vi "智能锁模.vi"() -> ()   [LabVIEW 2017]
panel:
  out "波形图表":dbl[](graph)=[-0.6363858363858363, -0.6363858363858363, -0.6490842490842491, 0.5611721611721612, 0.5142857142857142, 0.4586080586080586, 0.398046398046398, 0.32967032967032966, 0.2564102564102564, 0.1772893772893773, 0.09816849816849817, 0.016117216117216115, -0.06593406593406594, -0.147985347985348, -0.22417582417582418, -0.2993894993894994, -0.3716727716727717, -0.4332112332112332, -0.4918192918192918, -0.5416361416361416, -0.5826617826617827, -0.6148962148962149, -0.6363858363858363, -0.6490842490842491, -0.652014652014652, -0.6422466422466423, -0.6236874236874237, -0.5973137973137973, -0.5582417582417583, -0.5123321123321123, -0.45665445665445664, -0.3941391941391941, -0.32576312576312577, -0.2525030525030525, -0.17533577533577532, -0.09328449328449329, -0.014163614163614164, 0.06788766788766788, 0.14896214896214896, 0.2271062271062271, 0.3023199023199023, 0.3716727716727717, 0.43614163614163615, 0.4937728937728938, 0.5445665445665445, 0.5846153846153846, 0.6178266178266179, 0.6383394383394383, 0.652014652014652, 0.652014652014652, 0.6432234432234433, 0.6266178266178266, 0.5982905982905983, 0.5592185592185592, 0.5142857142857142, 0.45958485958485956, 0.39706959706959705, 0.3286935286935287, 0.2554334554334554, 0.17826617826617827, 0.09816849816849817, 0.017094017094017096, -0.06593406593406594, -0.147008547008547, -0.22612942612942613, -0.30036630036630035, -0.3716727716727717, -0.4341880341880342, -0.4918192918192918, -0.5426129426129426, -0.5836385836385837, -0.613919413919414, -0.6373626373626373, -0.6481074481074481, -0.652014652014652, -0.6442002442002442, -0.6246642246642247, -0.5963369963369963, -0.5572649572649573, -0.5103785103785103, -0.45567765567765567, -0.3941391941391941, -0.32673992673992674, -0.2515262515262515, -0.17631257631257632, -0.09523809523809523, -0.013186813186813187, 0.06788766788766788, 0.147985347985348, 0.2271062271062271, 0.3023199023199023, 0.3716727716727717, 0.43614163614163615, 0.49572649572649574, 0.5435897435897435, 0.5846153846153846, 0.6178266178266179, 0.6383394383394383, 0.652014652014652, 0.652991452991453, 0.6461538461538462, 0.6266178266178266, 0.5992673992673992, 0.5601953601953602, 0.5123321123321123, 0.45958485958485956, 0.39706959706959705, 0.32967032967032966, 0.25445665445665444, 0.1772893772893773, 0.0971916971916972, 0.016117216117216115, -0.06691086691086691, -0.147008547008547, -0.22515262515262516, -0.30036630036630035, -0.3706959706959707, -0.4341880341880342, -0.4908424908424908, -0.5416361416361416, -0.5816849816849817, -0.6148962148962149, -0.6363858363858363, -0.6500610500610501, -0.6510378510378511, -0.6422466422466423, -0.6246642246642247, -0.5982905982905983, -0.5582417582417583, -0.5103785103785103, -0.45665445665445664, -0.39706959706959705, -0.3277167277167277, -0.2515262515262515, -0.17631257631257632, -0.0971916971916972, -0.01514041514041514, 0.06788766788766788, 0.14896214896214896, 0.22612942612942613, 0.3013431013431013, 0.3716727716727717, 0.43614163614163615, 0.4937728937728938, 0.5445665445665445, 0.5846153846153846, 0.6168498168498169, 0.6393162393162393, 0.6510378510378511, 0.653968253968254, 0.6451770451770452, 0.6256410256410256, 0.5973137973137973, 0.5601953601953602, 0.5142857142857142, 0.4576312576312576, 0.39706959706959705, 0.32673992673992674, 0.25445665445665444, 0.17631257631257632, 0.09816849816849817, 0.016117216117216115, -0.06593406593406594, -0.147985347985348, -0.22515262515262516, -0.2993894993894994, -0.36874236874236876, -0.4341880341880342, -0.4937728937728938, -0.5426129426129426, -0.5807081807081808, -0.6158730158730159, -0.6363858363858363, -0.6500610500610501, -0.6500610500610501, -0.6432234432234433, -0.6236874236874237, -0.5953601953601954, -0.5572649572649573, -0.5113553113553113, -0.45665445665445664, -0.3941391941391941, -0.32673992673992674, -0.25347985347985347, -0.17631257631257632, -0.09426129426129426, -0.01221001221001221, 0.06788766788766788, 0.147985347985348, 0.22612942612942613, 0.3023199023199023, 0.37362637362637363, 0.4351648351648352, 0.4937728937728938, 0.5435897435897435, 0.5836385836385837, 0.6168498168498169, 0.6373626373626373, 0.6500610500610501, 0.652014652014652, 0.6442002442002442, 0.6266178266178266, 0.5992673992673992, 0.5592185592185592, 0.5133089133089133, 0.46056166056166054, 0.39706959706959705, 0.3286935286935287, 0.25445665445665444, 0.17826617826617827, 0.09816849816849817, 0.016117216117216115, -0.06593406593406594, -0.147008547008547, -0.22515262515262516, -0.30036630036630035, -0.3706959706959707, -0.4351648351648352, -0.4918192918192918, -0.5416361416361416, -0.5836385836385837, -0.6158730158730159, -0.6373626373626373, -0.6510378510378511, -0.652014652014652, -0.6432234432234433, -0.6227106227106227, -0.5973137973137973, -0.5572649572649573, -0.5113553113553113, -0.45567765567765567, -0.3951159951159951, -0.32576312576312577, -0.25347985347985347, -0.17631257631257632, -0.09621489621489622, -0.014163614163614164, 0.06691086691086691, 0.14896214896214896, 0.22612942612942613, 0.3013431013431013, 0.37362637362637363, 0.43614163614163615, 0.4927960927960928, 0.5435897435897435, 0.5846153846153846, 0.6168498168498169, 0.6393162393162393, 0.652014652014652, 0.652014652014652, 0.6451770451770452, 0.6256410256410256, 0.5973137973137973, 0.5592185592185592, 0.5142857142857142, 0.45958485958485956, 0.3960927960927961, 0.3286935286935287, 0.25445665445665444, 0.17826617826617827, 0.0971916971916972, 0.016117216117216115, -0.06691086691086691, -0.14603174603174604, -0.22515262515262516, -0.2993894993894994, -0.3706959706959707, -0.4332112332112332, -0.4918192918192918, -0.5406593406593406, -0.5816849816849817, -0.6158730158730159, -0.6363858363858363, -0.6490842490842491, -0.6510378510378511, -0.6422466422466423, -0.6246642246642247, -0.5963369963369963, -0.5582417582417583, -0.5103785103785103, -0.45665445665445664, -0.3941391941391941, -0.3277167277167277, -0.2525030525030525, -0.17533577533577532, -0.09621489621489622, -0.013186813186813187, 0.06788766788766788, 0.147008547008547, 0.2271062271062271, 0.3023199023199023, 0.3716727716727717, 0.4371184371184371, 0.4918192918192918, 0.5426129426129426, 0.5846153846153846, 0.6178266178266179, 0.6393162393162393, 0.6500610500610501, 0.652014652014652, 0.6442002442002442, 0.6256410256410256, 0.5992673992673992, 0.5601953601953602, 0.5133089133089133, 0.4586080586080586, 0.39706959706959705, 0.3277167277167277, 0.25445665445665444, 0.17826617826617827, 0.0971916971916972, 0.016117216117216115, -0.06398046398046398, -0.147008547008547, -0.22417582417582418, -0.2984126984126984, -0.3706959706959707, -0.4341880341880342, -0.4927960927960928, -0.5426129426129426, -0.5816849816849817, -0.6148962148962149, -0.6373626373626373, -0.6500610500610501, -0.6500610500610501, -0.6422466422466423, -0.6236874236874237, -0.5963369963369963, -0.5582417582417583, -0.5113553113553113, -0.45567765567765567, -0.3951159951159951, -0.32673992673992674, -0.2515262515262515, -0.1772893772893773, -0.09426129426129426, -0.01514041514041514, 0.06886446886446887, 0.147985347985348, 0.22612942612942613, 0.3013431013431013, 0.3706959706959707, 0.4380952380952381, 0.4937728937728938, 0.5445665445665445, 0.5836385836385837, 0.6178266178266179, 0.6373626373626373, 0.652014652014652, 0.652014652014652, 0.6442002442002442, 0.6256410256410256, 0.5973137973137973, 0.5611721611721612, 0.5152625152625152, 0.4586080586080586, 0.3960927960927961, 0.3277167277167277, 0.25445665445665444, 0.1772893772893773, 0.09816849816849817, 0.01514041514041514, -0.06593406593406594, -0.147008547008547, -0.22612942612942613, -0.2993894993894994, -0.3706959706959707, -0.4351648351648352, -0.4918192918192918, -0.5416361416361416, -0.5836385836385837, -0.6158730158730159, -0.6354090354090354, -0.6500610500610501, -0.6510378510378511, -0.6432234432234433, -0.6256410256410256, -0.5973137973137973, -0.5582417582417583, -0.5113553113553113, -0.45665445665445664, -0.3941391941391941, -0.32673992673992674, -0.2525030525030525, -0.17533577533577532, -0.09523809523809523, -0.014163614163614164, 0.06788766788766788, 0.147985347985348, 0.22612942612942613, 0.3023199023199023, 0.37264957264957266, 0.4371184371184371, 0.4937728937728938, 0.5435897435897435, 0.5836385836385837, 0.6178266178266179, 0.6393162393162393, 0.6510378510378511, 0.653968253968254, 0.6432234432234433, 0.6236874236874237, 0.5973137973137973, 0.5592185592185592, 0.5133089133089133, 0.4586080586080586, 0.3960927960927961, 0.3286935286935287, 0.25347985347985347, 0.1772893772893773, 0.0971916971916972, 0.016117216117216115, -0.06691086691086691, -0.147008547008547, -0.22515262515262516, -0.30036630036630035, -0.36971916971916974, -0.4341880341880342, -0.4927960927960928, -0.5426129426129426, -0.5836385836385837, -0.613919413919414, -0.6354090354090354, -0.652014652014652, -0.6490842490842491, -0.6432234432234433, -0.6236874236874237, -0.5953601953601954, -0.5572649572649573, -0.5103785103785103, -0.45665445665445664, -0.3960927960927961, -0.32576312576312577, -0.25347985347985347, -0.17435897435897435, -0.09621489621489622, -0.014163614163614164, 0.06788766788766788, 0.14896214896214896, 0.22612942612942613, 0.3032967032967033, 0.37362637362637363, 0.43614163614163615, 0.49474969474969477, 0.5435897435897435, 0.5855921855921856, 0.6178266178266179, 0.6373626373626373, 0.6510378510378511, 0.653968253968254, 0.6461538461538462, 0.6266178266178266, 0.5963369963369963, 0.5582417582417583, 0.5152625152625152, 0.45958485958485956, 0.3960927960927961, 0.3277167277167277, 0.2564102564102564, 0.17826617826617827, 0.0971916971916972, 0.016117216117216115, -0.06593406593406594, -0.147985347985348, -0.22612942612942613, -0.2993894993894994, -0.3706959706959707, -0.4341880341880342, -0.4908424908424908, -0.5426129426129426, -0.5807081807081808, -0.6148962148962149, -0.6363858363858363, -0.6510378510378511, -0.6490842490842491, -0.6412698412698413, -0.6236874236874237, -0.5943833943833944, -0.5582417582417583, -0.5103785103785103, -0.45567765567765567, -0.3941391941391941, -0.32673992673992674, -0.2525030525030525, -0.17631257631257632, -0.09426129426129426, -0.014163614163614164, 0.06691086691086691, 0.14896214896214896, 0.22612942612942613, 0.3023199023199023, 0.37362637362637363, 0.4371184371184371, 0.4927960927960928, 0.5445665445665445, 0.5846153846153846, 0.6178266178266179, 0.6373626373626373, 0.652014652014652, 0.653968253968254, 0.6451770451770452, 0.6256410256410256, 0.5982905982905983, 0.5601953601953602, 0.5133089133089133, 0.4586080586080586, 0.3960927960927961, 0.3286935286935287, 0.25347985347985347, 0.17924297924297924]
  out "数组":dbl[](array[numeric])=[-0.6363858363858363, -0.6363858363858363, -0.6490842490842491, 0.5611721611721612, 0.5142857142857142, 0.4586080586080586, 0.398046398046398, 0.32967032967032966, 0.2564102564102564, 0.1772893772893773, 0.09816849816849817, 0.016117216117216115, -0.06593406593406594, -0.147985347985348, -0.22417582417582418, -0.2993894993894994, -0.3716727716727717, -0.4332112332112332, -0.4918192918192918, -0.5416361416361416, -0.5826617826617827, -0.6148962148962149, -0.6363858363858363, -0.6490842490842491, -0.652014652014652, -0.6422466422466423, -0.6236874236874237, -0.5973137973137973, -0.5582417582417583, -0.5123321123321123, -0.45665445665445664, -0.3941391941391941, -0.32576312576312577, -0.2525030525030525, -0.17533577533577532, -0.09328449328449329, -0.014163614163614164, 0.06788766788766788, 0.14896214896214896, 0.2271062271062271, 0.3023199023199023, 0.3716727716727717, 0.43614163614163615, 0.4937728937728938, 0.5445665445665445, 0.5846153846153846, 0.6178266178266179, 0.6383394383394383, 0.652014652014652, 0.652014652014652, 0.6432234432234433, 0.6266178266178266, 0.5982905982905983, 0.5592185592185592, 0.5142857142857142, 0.45958485958485956, 0.39706959706959705, 0.3286935286935287, 0.2554334554334554, 0.17826617826617827, 0.09816849816849817, 0.017094017094017096, -0.06593406593406594, -0.147008547008547, -0.22612942612942613, -0.30036630036630035, -0.3716727716727717, -0.4341880341880342, -0.4918192918192918, -0.5426129426129426, -0.5836385836385837, -0.613919413919414, -0.6373626373626373, -0.6481074481074481, -0.652014652014652, -0.6442002442002442, -0.6246642246642247, -0.5963369963369963, -0.5572649572649573, -0.5103785103785103, -0.45567765567765567, -0.3941391941391941, -0.32673992673992674, -0.2515262515262515, -0.17631257631257632, -0.09523809523809523, -0.013186813186813187, 0.06788766788766788, 0.147985347985348, 0.2271062271062271, 0.3023199023199023, 0.3716727716727717, 0.43614163614163615, 0.49572649572649574, 0.5435897435897435, 0.5846153846153846, 0.6178266178266179, 0.6383394383394383, 0.652014652014652, 0.652991452991453, 0.6461538461538462, 0.6266178266178266, 0.5992673992673992, 0.5601953601953602, 0.5123321123321123, 0.45958485958485956, 0.39706959706959705, 0.32967032967032966, 0.25445665445665444, 0.1772893772893773, 0.0971916971916972, 0.016117216117216115, -0.06691086691086691, -0.147008547008547, -0.22515262515262516, -0.30036630036630035, -0.3706959706959707, -0.4341880341880342, -0.4908424908424908, -0.5416361416361416, -0.5816849816849817, -0.6148962148962149, -0.6363858363858363, -0.6500610500610501, -0.6510378510378511, -0.6422466422466423, -0.6246642246642247, -0.5982905982905983, -0.5582417582417583, -0.5103785103785103, -0.45665445665445664, -0.39706959706959705, -0.3277167277167277, -0.2515262515262515, -0.17631257631257632, -0.0971916971916972, -0.01514041514041514, 0.06788766788766788, 0.14896214896214896, 0.22612942612942613, 0.3013431013431013, 0.3716727716727717, 0.43614163614163615, 0.4937728937728938, 0.5445665445665445, 0.5846153846153846, 0.6168498168498169, 0.6393162393162393, 0.6510378510378511, 0.653968253968254, 0.6451770451770452, 0.6256410256410256, 0.5973137973137973, 0.5601953601953602, 0.5142857142857142, 0.4576312576312576, 0.39706959706959705, 0.32673992673992674, 0.25445665445665444, 0.17631257631257632, 0.09816849816849817, 0.016117216117216115, -0.06593406593406594, -0.147985347985348, -0.22515262515262516, -0.2993894993894994, -0.36874236874236876, -0.4341880341880342, -0.4937728937728938, -0.5426129426129426, -0.5807081807081808, -0.6158730158730159, -0.6363858363858363, -0.6500610500610501, -0.6500610500610501, -0.6432234432234433, -0.6236874236874237, -0.5953601953601954, -0.5572649572649573, -0.5113553113553113, -0.45665445665445664, -0.3941391941391941, -0.32673992673992674, -0.25347985347985347, -0.17631257631257632, -0.09426129426129426, -0.01221001221001221, 0.06788766788766788, 0.147985347985348, 0.22612942612942613, 0.3023199023199023, 0.37362637362637363, 0.4351648351648352, 0.4937728937728938, 0.5435897435897435, 0.5836385836385837, 0.6168498168498169, 0.6373626373626373, 0.6500610500610501, 0.652014652014652, 0.6442002442002442, 0.6266178266178266, 0.5992673992673992, 0.5592185592185592, 0.5133089133089133, 0.46056166056166054, 0.39706959706959705, 0.3286935286935287, 0.25445665445665444, 0.17826617826617827, 0.09816849816849817, 0.016117216117216115, -0.06593406593406594, -0.147008547008547, -0.22515262515262516, -0.30036630036630035, -0.3706959706959707, -0.4351648351648352, -0.4918192918192918, -0.5416361416361416, -0.5836385836385837, -0.6158730158730159, -0.6373626373626373, -0.6510378510378511, -0.652014652014652, -0.6432234432234433, -0.6227106227106227, -0.5973137973137973, -0.5572649572649573, -0.5113553113553113, -0.45567765567765567, -0.3951159951159951, -0.32576312576312577, -0.25347985347985347, -0.17631257631257632, -0.09621489621489622, -0.014163614163614164, 0.06691086691086691, 0.14896214896214896, 0.22612942612942613, 0.3013431013431013, 0.37362637362637363, 0.43614163614163615, 0.4927960927960928, 0.5435897435897435, 0.5846153846153846, 0.6168498168498169, 0.6393162393162393, 0.652014652014652, 0.652014652014652, 0.6451770451770452, 0.6256410256410256, 0.5973137973137973, 0.5592185592185592, 0.5142857142857142, 0.45958485958485956, 0.3960927960927961, 0.3286935286935287, 0.25445665445665444, 0.17826617826617827, 0.0971916971916972, 0.016117216117216115, -0.06691086691086691, -0.14603174603174604, -0.22515262515262516, -0.2993894993894994, -0.3706959706959707, -0.4332112332112332, -0.4918192918192918, -0.5406593406593406, -0.5816849816849817, -0.6158730158730159, -0.6363858363858363, -0.6490842490842491, -0.6510378510378511, -0.6422466422466423, -0.6246642246642247, -0.5963369963369963, -0.5582417582417583, -0.5103785103785103, -0.45665445665445664, -0.3941391941391941, -0.3277167277167277, -0.2525030525030525, -0.17533577533577532, -0.09621489621489622, -0.013186813186813187, 0.06788766788766788, 0.147008547008547, 0.2271062271062271, 0.3023199023199023, 0.3716727716727717, 0.4371184371184371, 0.4918192918192918, 0.5426129426129426, 0.5846153846153846, 0.6178266178266179, 0.6393162393162393, 0.6500610500610501, 0.652014652014652, 0.6442002442002442, 0.6256410256410256, 0.5992673992673992, 0.5601953601953602, 0.5133089133089133, 0.4586080586080586, 0.39706959706959705, 0.3277167277167277, 0.25445665445665444, 0.17826617826617827, 0.0971916971916972, 0.016117216117216115, -0.06398046398046398, -0.147008547008547, -0.22417582417582418, -0.2984126984126984, -0.3706959706959707, -0.4341880341880342, -0.4927960927960928, -0.5426129426129426, -0.5816849816849817, -0.6148962148962149, -0.6373626373626373, -0.6500610500610501, -0.6500610500610501, -0.6422466422466423, -0.6236874236874237, -0.5963369963369963, -0.5582417582417583, -0.5113553113553113, -0.45567765567765567, -0.3951159951159951, -0.32673992673992674, -0.2515262515262515, -0.1772893772893773, -0.09426129426129426, -0.01514041514041514, 0.06886446886446887, 0.147985347985348, 0.22612942612942613, 0.3013431013431013, 0.3706959706959707, 0.4380952380952381, 0.4937728937728938, 0.5445665445665445, 0.5836385836385837, 0.6178266178266179, 0.6373626373626373, 0.652014652014652, 0.652014652014652, 0.6442002442002442, 0.6256410256410256, 0.5973137973137973, 0.5611721611721612, 0.5152625152625152, 0.4586080586080586, 0.3960927960927961, 0.3277167277167277, 0.25445665445665444, 0.1772893772893773, 0.09816849816849817, 0.01514041514041514, -0.06593406593406594, -0.147008547008547, -0.22612942612942613, -0.2993894993894994, -0.3706959706959707, -0.4351648351648352, -0.4918192918192918, -0.5416361416361416, -0.5836385836385837, -0.6158730158730159, -0.6354090354090354, -0.6500610500610501, -0.6510378510378511, -0.6432234432234433, -0.6256410256410256, -0.5973137973137973, -0.5582417582417583, -0.5113553113553113, -0.45665445665445664, -0.3941391941391941, -0.32673992673992674, -0.2525030525030525, -0.17533577533577532, -0.09523809523809523, -0.014163614163614164, 0.06788766788766788, 0.147985347985348, 0.22612942612942613, 0.3023199023199023, 0.37264957264957266, 0.4371184371184371, 0.4937728937728938, 0.5435897435897435, 0.5836385836385837, 0.6178266178266179, 0.6393162393162393, 0.6510378510378511, 0.653968253968254, 0.6432234432234433, 0.6236874236874237, 0.5973137973137973, 0.5592185592185592, 0.5133089133089133, 0.4586080586080586, 0.3960927960927961, 0.3286935286935287, 0.25347985347985347, 0.1772893772893773, 0.0971916971916972, 0.016117216117216115, -0.06691086691086691, -0.147008547008547, -0.22515262515262516, -0.30036630036630035, -0.36971916971916974, -0.4341880341880342, -0.4927960927960928, -0.5426129426129426, -0.5836385836385837, -0.613919413919414, -0.6354090354090354, -0.652014652014652, -0.6490842490842491, -0.6432234432234433, -0.6236874236874237, -0.5953601953601954, -0.5572649572649573, -0.5103785103785103, -0.45665445665445664, -0.3960927960927961, -0.32576312576312577, -0.25347985347985347, -0.17435897435897435, -0.09621489621489622, -0.014163614163614164, 0.06788766788766788, 0.14896214896214896, 0.22612942612942613, 0.3032967032967033, 0.37362637362637363, 0.43614163614163615, 0.49474969474969477, 0.5435897435897435, 0.5855921855921856, 0.6178266178266179, 0.6373626373626373, 0.6510378510378511, 0.653968253968254, 0.6461538461538462, 0.6266178266178266, 0.5963369963369963, 0.5582417582417583, 0.5152625152625152, 0.45958485958485956, 0.3960927960927961, 0.3277167277167277, 0.2564102564102564, 0.17826617826617827, 0.0971916971916972, 0.016117216117216115, -0.06593406593406594, -0.147985347985348, -0.22612942612942613, -0.2993894993894994, -0.3706959706959707, -0.4341880341880342, -0.4908424908424908, -0.5426129426129426, -0.5807081807081808, -0.6148962148962149, -0.6363858363858363, -0.6510378510378511, -0.6490842490842491, -0.6412698412698413, -0.6236874236874237, -0.5943833943833944, -0.5582417582417583, -0.5103785103785103, -0.45567765567765567, -0.3941391941391941, -0.32673992673992674, -0.2525030525030525, -0.17631257631257632, -0.09426129426129426, -0.014163614163614164, 0.06691086691086691, 0.14896214896214896, 0.22612942612942613, 0.3023199023199023, 0.37362637362637363, 0.4371184371184371, 0.4927960927960928, 0.5445665445665445, 0.5846153846153846, 0.6178266178266179, 0.6373626373626373, 0.652014652014652, 0.653968253968254, 0.6451770451770452, 0.6256410256410256, 0.5982905982905983, 0.5601953601953602, 0.5133089133089133, 0.4586080586080586, 0.3960927960927961, 0.3286935286935287, 0.25347985347985347, 0.17924297924297924]
  out "数据输出":string
  in  "选项卡控件":enum32{"UDP协议", "AD读取", "DA控制"}(tab)=enum."AD读取"
  in  "AD地址":string="191.168.1.10"
  in  "本地端口":u16=1234
  in  "DA地址":string="192.168.1.2"
  in  "停止":bool
  in  "远程端口":u16=1234
  in  "采集最大值（byte）":u16=1020
  in  "读取":bool
  in  "DA1数值":dbl min=-5.0 max=5.0 format="%.3f"
  out "发送字符串":string
  in  "DA2数值":dbl min=-5.0 max=5.0 format="%.3f"
  in  "DA3数值":dbl min=-5.0 max=5.0 format="%.3f"
  in  "DA4数值":dbl=1.0 min=-5.0 max=5.0 format="%.3f"
  in  "最低电压":dbl=-5.0
  in  "最高电压":dbl=5.0
  in  "电压精度":u8=14
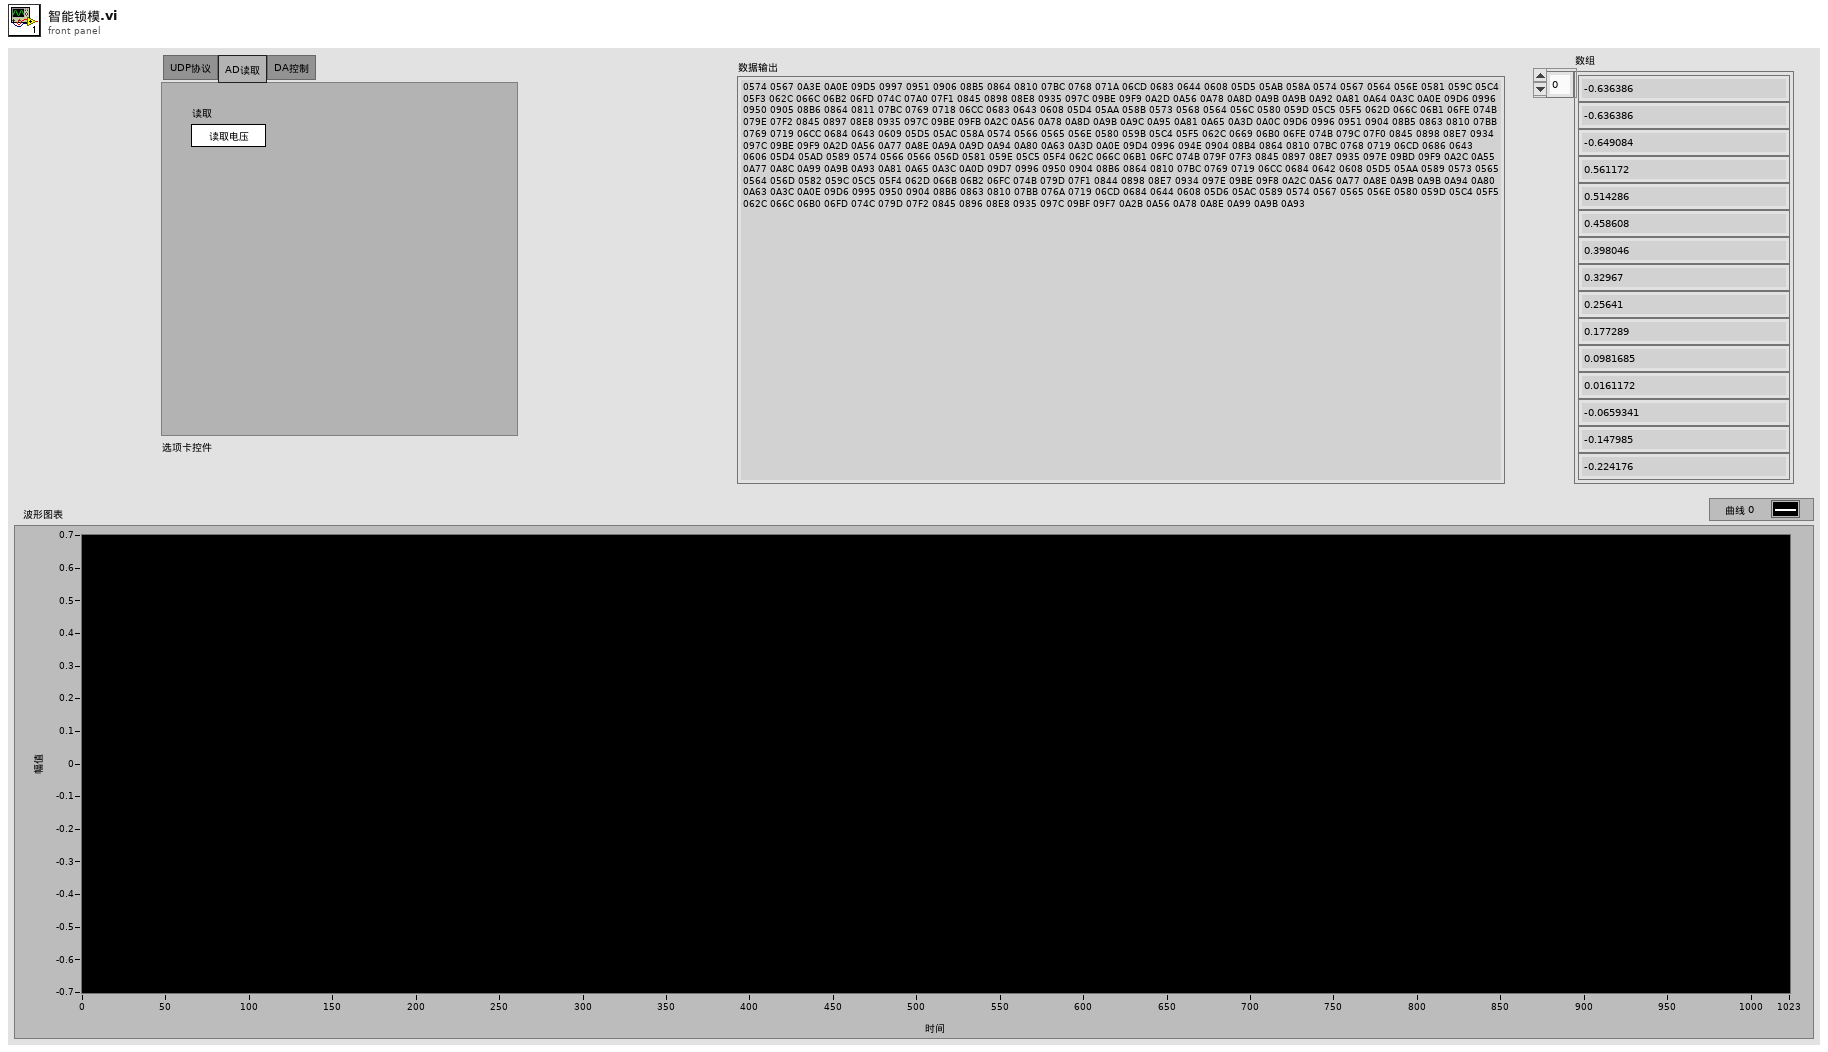
[diagram p1: front panel]
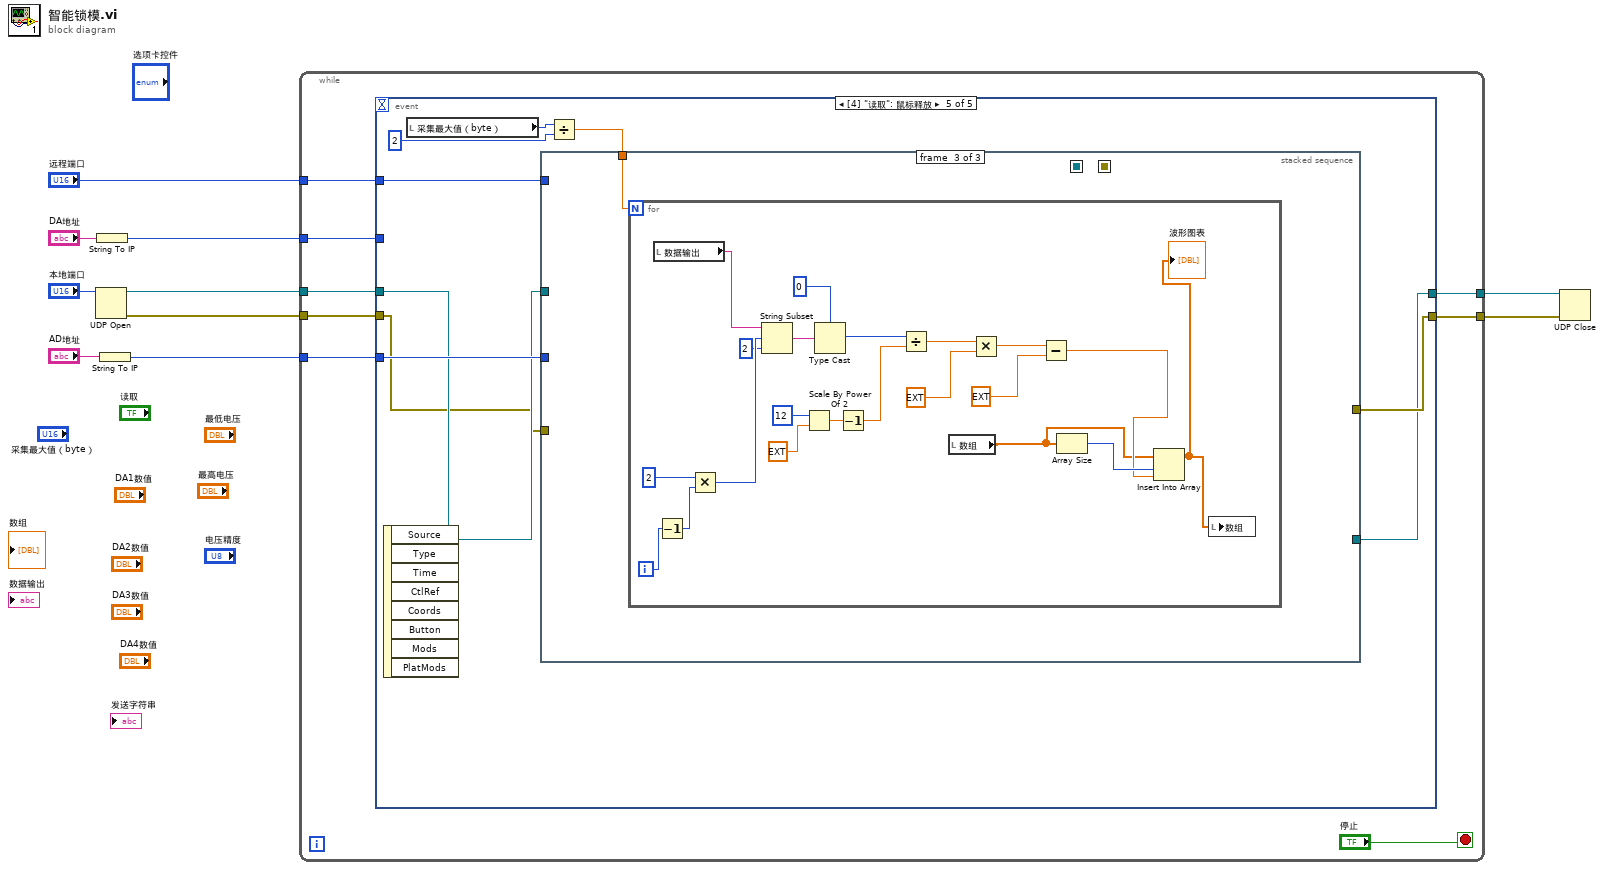
[diagram p0: block diagram]
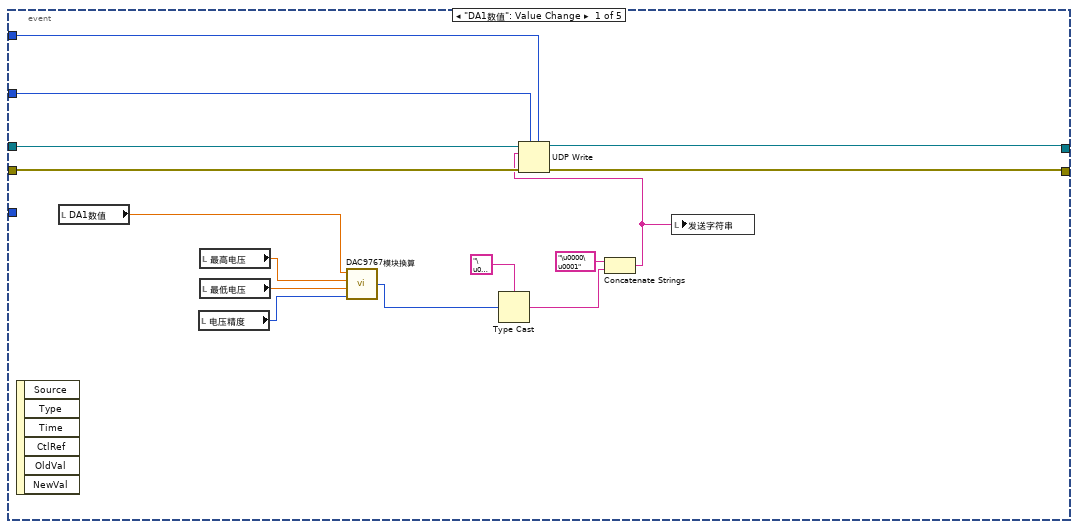
[diagram p2: hidden frame]
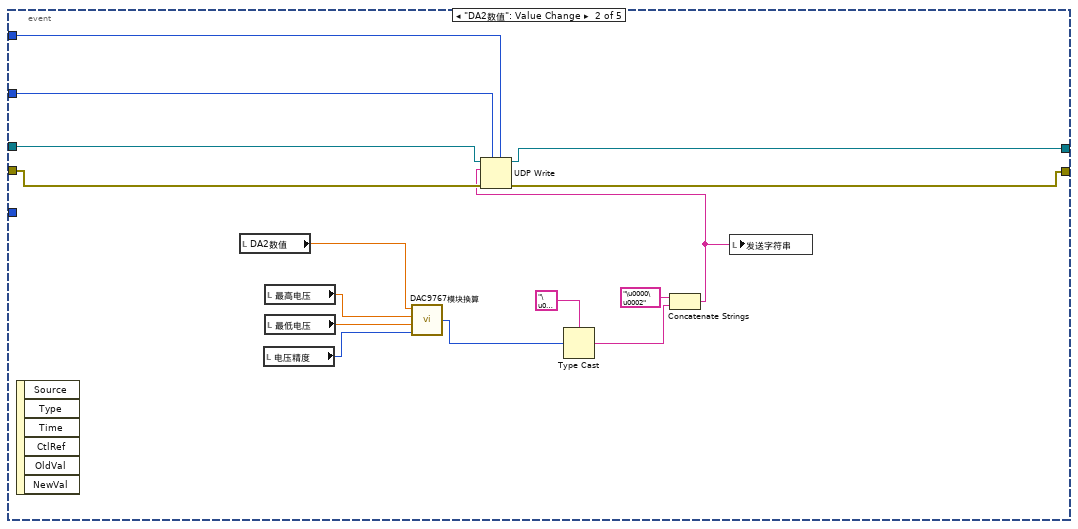
[diagram p3: hidden frame]
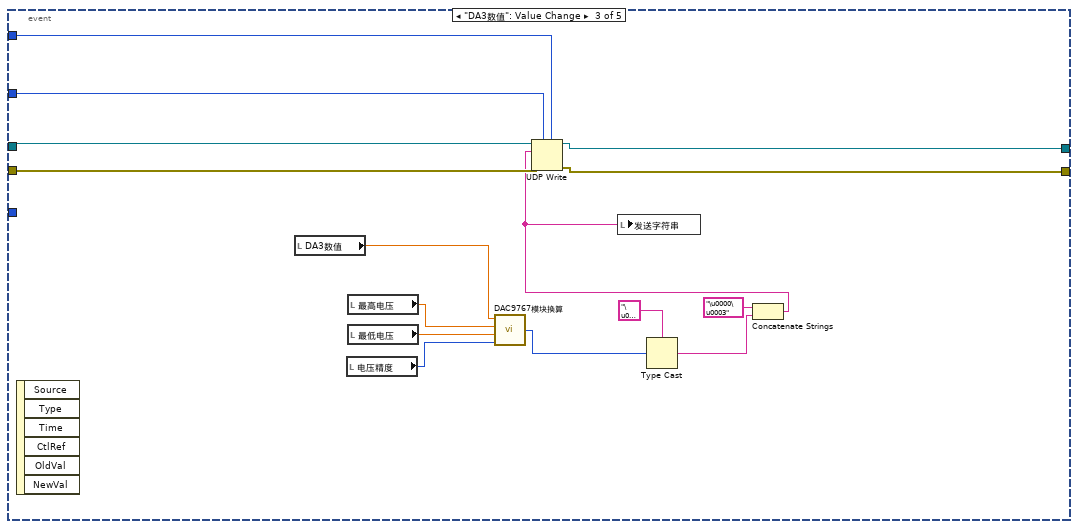
[diagram p4: hidden frame]
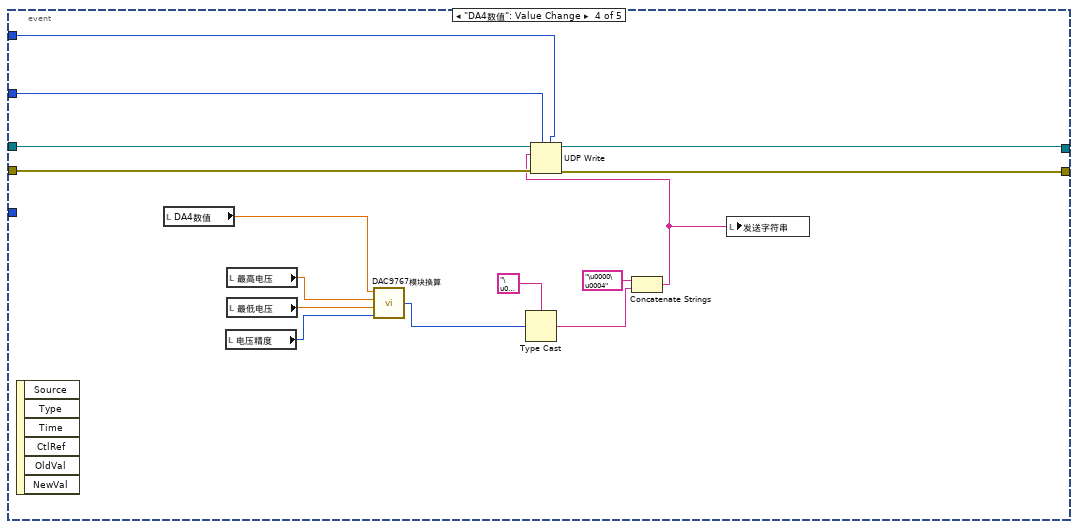
[diagram p5: hidden frame]
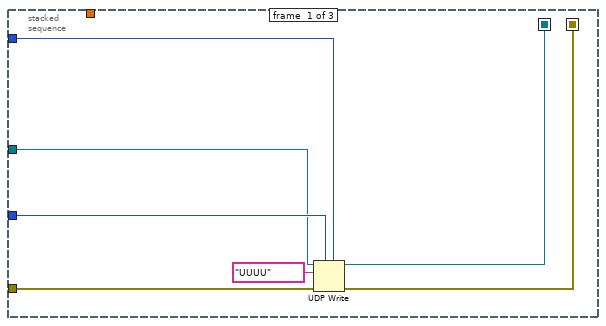
[diagram p6: hidden frame]
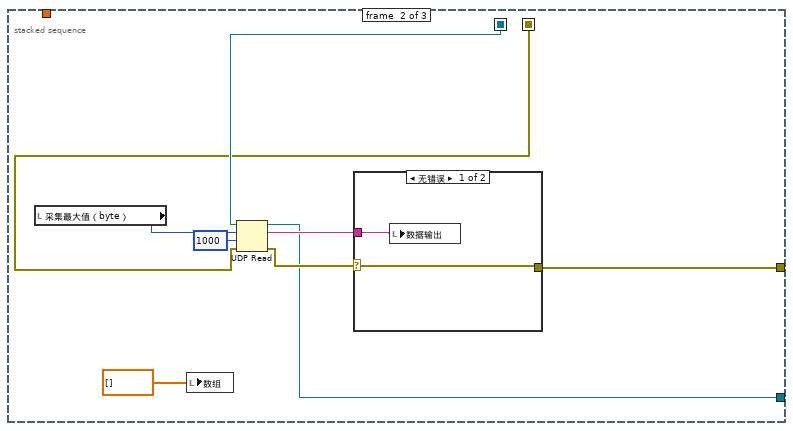
[diagram p7: hidden frame]
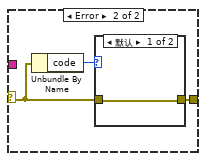
[diagram p8: hidden frame]
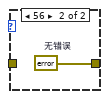
[diagram p9: hidden frame]
diagram:
  n1 = UDP Open(11:"本地端口") -> (port=w6:refnum<k16>, 0:w5:errorcluster)  [unwired: 4 in, 1 out]
  n2 = String To IP(1:"DA地址") -> (0:w9:u32)
  n3 = String To IP(1:"AD地址") -> (0:w1:u32)
  n4 = while {
    tunnel: w6 -> [w18]
    tunnel: w5 -> [w17]
    tunnel: w9 -> [w16]
    tunnel: [w14] -> w3
    tunnel: [w13] -> w4
    tunnel: "远程端口" -> [w12]
    tunnel: w1 -> [w11]
    stop <- "停止" stop-if-true
    n5 = event shown="[4] \"读取\": 鼠标释放" {
      selector: _ -> [_ _ _ _ _]
      dyn-events: _ -> [_ _ _ _ _]
      timeout: _ -> [_ _ _ _ _]
      tunnel: w18 -> [w28 w41 w56 w71 w85]
      tunnel: w17 -> [w30 w40 w55 w70 w84]
      tunnel: w16 -> [w29 w36 w54 w69 _]
      tunnel: [w33 w39 w52 w67 w82] -> w14
      tunnel: [w32 w38 w51 w66 w83] -> w13
      tunnel: w12 -> [w31 w37 w53 w68 w86]
      tunnel: w11 -> [_ _ _ _ w87]
      event "DA1数值": Value Change {
        n6 = event-data() -> ()  [unwired: 1 in, 6 out]
        n7 = local read "DA1数值"() -> (w24:dbl)
        n8 = local read "电压精度"() -> (w20:u8)
        n9 = local read "最高电压"() -> (w21:dbl)
        n10 = local read "最低电压"() -> (w22:dbl)
        n11 = call "DAC9767模块换算.vi"("电压精度"=w20, "最低电压"=w22, "最高电压"=w21, "数值"=w24) -> ("换算16进制"=w23:u16)
        n12 = Type Cast(type="\u0001" ("类型"), x=w23) -> (*(type *) &x=w25:string)
        n13 = Concatenate Strings("\u0000\u0001" ("字符串"), w25) -> (w19:string)
        n14 = UDP Write(address=w29, port or service name=w31, connection ID=w28, data in=w19, 8:w30) -> (error out=w32:errorcluster, 3:w33:refnum<k16>)  [unwired: 1 in]
        n15 = local write "发送字符串"(w19) -> ()
      }
      event "DA2数值": Value Change {
        n16 = event-data() -> ()  [unwired: 1 in, 6 out]
        n17 = local read "DA2数值"() -> (w35:dbl)
        n18 = local read "电压精度"() -> (w42:u8)
        n19 = local read "最高电压"() -> (w43:dbl)
        n20 = local read "最低电压"() -> (w44:dbl)
        n21 = call "DAC9767模块换算.vi"("电压精度"=w42, "最低电压"=w44, "最高电压"=w43, "数值"=w35) -> ("换算16进制"=w45:u16)
        n22 = Type Cast(type="\u0001" ("类型"), x=w45) -> (*(type *) &x=w46:string)
        n23 = Concatenate Strings("\u0000\u0002" ("字符串"), w46) -> (w34:string)
        n24 = UDP Write(address=w36, port or service name=w37, connection ID=w41, data in=w34, 8:w40) -> (error out=w38:errorcluster, 3:w39:refnum<k16>)  [unwired: 1 in]
        n25 = local write "发送字符串"(w34) -> ()
      }
      event "DA3数值": Value Change {
        n26 = event-data() -> ()  [unwired: 1 in, 6 out]
        n27 = local read "DA3数值"() -> (w50:dbl)
        n28 = local read "电压精度"() -> (w57:u8)
        n29 = local read "最高电压"() -> (w58:dbl)
        n30 = local read "最低电压"() -> (w59:dbl)
        n31 = call "DAC9767模块换算.vi"("电压精度"=w57, "最低电压"=w59, "最高电压"=w58, "数值"=w50) -> ("换算16进制"=w60:u16)
        n32 = Type Cast(type="\u0001" ("类型"), x=w60) -> (*(type *) &x=w61:string)
        n33 = Concatenate Strings("\u0000\u0003" ("字符串"), w61) -> (w49:string)
        n34 = UDP Write(address=w54, port or service name=w53, connection ID=w56, data in=w49, 8:w55) -> (error out=w51:errorcluster, 3:w52:refnum<k16>)  [unwired: 1 in]
        n35 = local write "发送字符串"(w49) -> ()
      }
      event "DA4数值": Value Change {
        n36 = event-data() -> ()  [unwired: 1 in, 6 out]
        n37 = local read "DA4数值"() -> (w65:dbl)
        n38 = local read "电压精度"() -> (w74:u8)
        n39 = local read "最高电压"() -> (w75:dbl)
        n40 = local read "最低电压"() -> (w76:dbl)
        n41 = call "DAC9767模块换算.vi"("电压精度"=w74, "最低电压"=w76, "最高电压"=w75, "数值"=w65) -> ("换算16进制"=w77:u16)
        n42 = Type Cast(type="\u0001" ("类型"), x=w77) -> (*(type *) &x=w78:string)
        n43 = Concatenate Strings("\u0000\u0004" ("字符串"), w78) -> (w64:string)
        n44 = UDP Write(address=w69, port or service name=w68, connection ID=w71, data in=w64, 8:w70) -> (error out=w66:errorcluster, 3:w67:refnum<k16>)  [unwired: 1 in]
        n45 = local write "发送字符串"(w64) -> ()
      }
      event "读取": Mouse Up {
        n46 = event-data() -> ()  [unwired: 1 in, 8 out]
        n47 = local read "采集最大值（byte）"() -> (w81:u16)
        n48 = Divide(x=w81, y=u16 2) -> (x/y=w79:dbl)
        n49 = stacked-sequence {
          seq-local: [w89 _ _] -> [_ w96 _]
          seq-local: [w88 _ _] -> [_ w95 _]
          tunnel: w87 -> [w94 _ _]
          tunnel: w86 -> [w93 _ _]
          tunnel: w85 -> [w92 _ _]
          tunnel: w84 -> [w91 _ _]
          tunnel: [_ w99 _] -> w83
          tunnel: [_ w98 _] -> w82
          tunnel: w79 -> [_ _ w111]
          frame #0 {
            n50 = UDP Write(address=w94, port or service name=w93, connection ID=w92, data in="UUUU" ("数据输入"), 8:w91) -> (error out=w88:errorcluster, 3:w89:refnum<k16>)  [unwired: 1 in]
          }
          frame #1 {
            n51 = local read "采集最大值（byte）"() -> (w103:u16)
            n52 = local write "数组"(dbl[] []) -> ()
            n53 = UDP Read(connection ID=w96, max size (548)=w103, timeout ms (25000)=1000 ("超时毫秒(25000)"), 8:w95) -> (data out=w101:string, error out=w100:errorcluster, 3:w98:refnum<k16>)  [unwired: 2 out]
            n54 = case shown="无错误" w100 {
              selector: w100 -> [w104 w107]
              tunnel: w101 -> [w105 _]
              tunnel: [w104 w106] -> w99
              frame No Error {
                n55 = local write "数据输出"(w105) -> ()
              }
              frame Error {
                n56 = Unbundle By Name(w107) -> ("code"=w108:i32)
                n57 = case shown="默认" w108 {
                  tunnel: w107 -> [w109 _]
                  tunnel: [w109 w110] -> w106
                  frame Default {
                  }
                  frame 56 {
                    w110 = errorcluster {"status"=FALSE, "code"=0, "source"=""}  # 无错误
                  }
                }
              }
            }
          }
          frame #2 {
            n58 = for {
              N: w111 -> [_]
              i -> [w128]
              n59 = local read "数据输出"() -> (w129:string)
              n60 = Decrement(x=w128) -> (x-1=w127:i32)
              n61 = Multiply(x=2, y=w127) -> (x*y=w131:i32)
              n62 = String Subset(string=w129, offset (0)=w131, length (rest)=2 ("长度（剩余）")) -> (substring=w126:string)
              n63 = Scale By Power Of 2(n=i16 12, x=ext 1.0) -> (x*2^n=w121:ext)
              n64 = Type Cast(type=u16 0, x=w126) -> (*(type *) &x=w124:u16)
              n65 = Decrement(x=w121) -> (x-1=w120:ext)
              n66 = Divide(x=w124, y=w120) -> (x/y=w119:ext)
              n67 = local read "数组"() -> (w113:dbl[])
              n68 = Multiply(x=w119, y=ext 4.0) -> (x*y=w117:ext)
              n69 = Subtract(x=w117, y=ext 2.0) -> (x-y=w114:ext)
              n70 = Array Size(array=w113) -> (size(s)=w115:i32)
              n71 = Insert Into Array(array=w113, index=w115, new element=w114) -> (w112:dbl[])
              "波形图表" <- w112
              n72 = local write "数组"(w112) -> ()
            }
          }
        }
      }
    }
  }
  n73 = UDP Close(connection ID=w3, 8:w4) -> ()  [unwired: 2 out]
